vi "Draw.vi"(8 "Error In":errorcluster, 11 "Pixel In":refnum<class "Square.lvclass">) -> (0 "Error Out":errorcluster, 2 "Element To Display":T1[](array[typedef]), 3 "Pixel Out":refnum<class "Square.lvclass">)   [LabVIEW 2019, in "Square.lvclass"]
uses:
  Square.lvclass
  C:/Users/goo13/Documents/GIT Local/myRIO-Neopixel/Source/RT/Display Element/Display Element.lvclass
  Display Element/Public/Controls/Pixel.ctl
  Display Element/Public/Controls/Vector.ctl
  Display Element/Display Element.lvclass
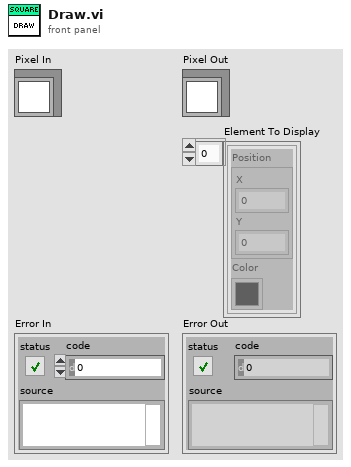
[diagram p1: front panel]
types:
  T1 = typedef "Display Element.lvclass/Pixel.ctl" = cluster{"Position":T2, "Color":u32}
  T2 = typedef "Display Element.lvclass/Vector.ctl" = cluster{"X":i32, "Y":i32}
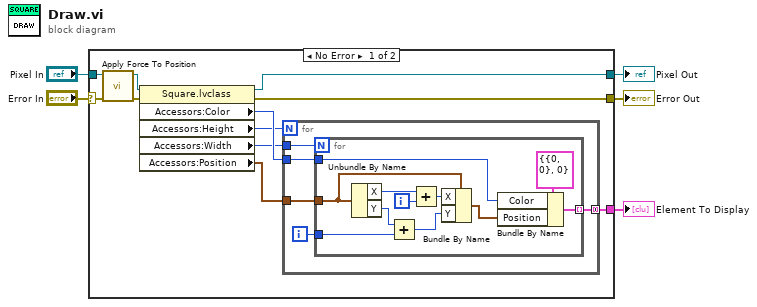
[diagram p0: block diagram]
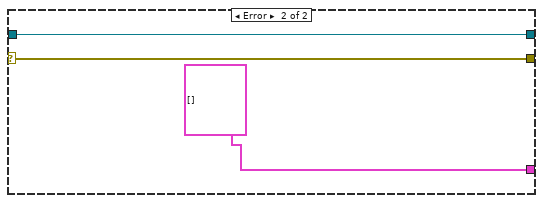
[diagram p2: hidden frame]
diagram:
  n1 = case shown="No Error" "Error In" {
    selector: "Error In" -> [w12 w35]
    tunnel: "Pixel In" -> [w11 w34]
    tunnel: [w15 w35] -> w3
    tunnel: [w16 w34] -> w2
    tunnel: [w13 T1[] []] -> w1
    frame No Error {
      n2 = call-dynamic "Apply Force To Position.vi"("Error In"=w12, "Display Element In"=w11) -> ("Error Out"=w10:errorcluster, "Display Element Out"=w9:refnum<class "Square.lvclass">)  [unwired: 8 in]
      n3 = property class="Square.lvclass"(reference=w9, error in=w10) -> (reference out=w16:refnum<class "Square.lvclass">, error out=w15:errorcluster, "Accessors:Color"=w14:u32, "Accessors:Height"=w8:u32, "Accessors:Width"=w7:u32, "Accessors:Position"=w6:T2)
      n4 = for {
        N: w8 -> [_]
        tunnel: w14 -> [w18]
        tunnel: [w17] -> w13 mode=concatenating
        tunnel: w7 -> [w21]
        tunnel: w6 -> [w20]
        i -> [w19]
        n5 = for {
          N: w21 -> [_]
          tunnel: w20 -> [w28]
          tunnel: w19 -> [w31]
          tunnel: w18 -> [w24]
          tunnel: [w23] -> w17 mode=indexing
          i -> [w29]
          n6 = Unbundle By Name(w28) -> ("X"=w30:i32, "Y"=w32:i32)
          n7 = Add(x=w32, y=w31) -> (x+y=w26:i32)
          n8 = Add(x=w30, y=w29) -> (x+y=w27:i32)
          n9 = Bundle By Name(cluster=w28, "X"=w27, "Y"=w26) -> (w22:T2)
          n10 = Bundle By Name(cluster=T1 {"Position"={"X"=0, "Y"=0}, "Color"=0} ("Pixel"), "Color"=w24, "Position"=w22) -> (w23:T1)
        }
      }
    }
    frame Error {
    }
  }
  "Pixel Out" <- w2
  "Error Out" <- w3
  "Element To Display" <- w1
